vi "OAT Manually Labeled Polar Plot.vi"(0 "picture":picture, 1 "picture \ndimensions (w,h)":cluster{"width":i16, "height":i16}, 2 "polar settings":T3={"polar attributes"={"maximum"=0.0, "minimum"=0.0, "clip to min"=FALSE, "log"=FALSE, "grid color"=3381657, "plot color"=16711680, "fmt and prec"={"format"=enum."Decimal", "precision"=1}, "visible section"=8}, "desired font(Application)"=enum."Application Font", "[user-specified font]"={"Font Name:"="", "Size"=0, "Strikeout?"=FALSE, "Italic?"=FALSE, "Underline?"=FALSE, "Outline?"=FALSE, "Shadow?"=FALSE, "Bold?"=FALSE}} {"polar attributes"."minimum" format="%.2f"; "polar attributes"."maximum" format="%.2f"}, 3 "cursor attributes":T6={"layout color"=852223, "active color"=16740820, "precision"=2, "BG transparent? (T)"=FALSE, "radius"=2}, 5 "magnitude":cluster{"X":dbl[], "Y":dbl[]} {"Y" format="%.2f"; "X" format="%.2f"}, 7 "phase lag(rad)":cluster{"X":dbl[], "Y":dbl[]} {"Y" format="%.2f"; "X" format="%.2f"}, 11 "error in (no error)":errorcluster, 12 "rotating settings":T2 {"shaft rotating direction" items=["CW", "CCW"]}, 13 "phase setting":T1) -> (4 "new picture":picture, 10 "Cursor List [EU Position] Out":T4(array[cluster]) {"Location"."Y" format="%.2f"; "Location"."X" format="%.2f"}, 15 "error out":errorcluster)   [LabVIEW 2017]
doc: "Draws a polar plot on a picture control that you can interactively label."
uses:
  <vilib>/addons/Sound and Vibration/Order Analysis/Backward Compatibility/SubVIs/OAT Polar Cursor Attributes.ctl
  <vilib>/addons/Sound and Vibration/Order Analysis/_OAT State Machine/OAT State Machine Generate Events for Booleans.vi
  <vilib>/addons/Sound and Vibration/Order Analysis/_OAT State Machine/OAT State Machine Generate Event for Numeric.vi
  <vilib>/addons/Sound and Vibration/Order Analysis/_OAT State Machine/OAT State Machine Generate Events for Numerics.vi
panel:
  in  "cursor":T5={"Name"="", "Color"=0, "Hair Style"=4, "Point Style"=2, "Name Visible"=TRUE, "Trackable"=TRUE, "Lock Style"=2, "Plot Number"=0, "Marker Index"=0, "Location"={"X"=0.5, "Y"=0.5}} {"Location"."Y" format="%.2f"; "Location"."X" format="%.2f"}
  in  "exit":bool
  in  "del cursor":bool
  in  "add cursor":bool
  out "XY Graph":cluster{"X":dbl[], "Y":dbl[]}(graph)
  out "polar plot":picture
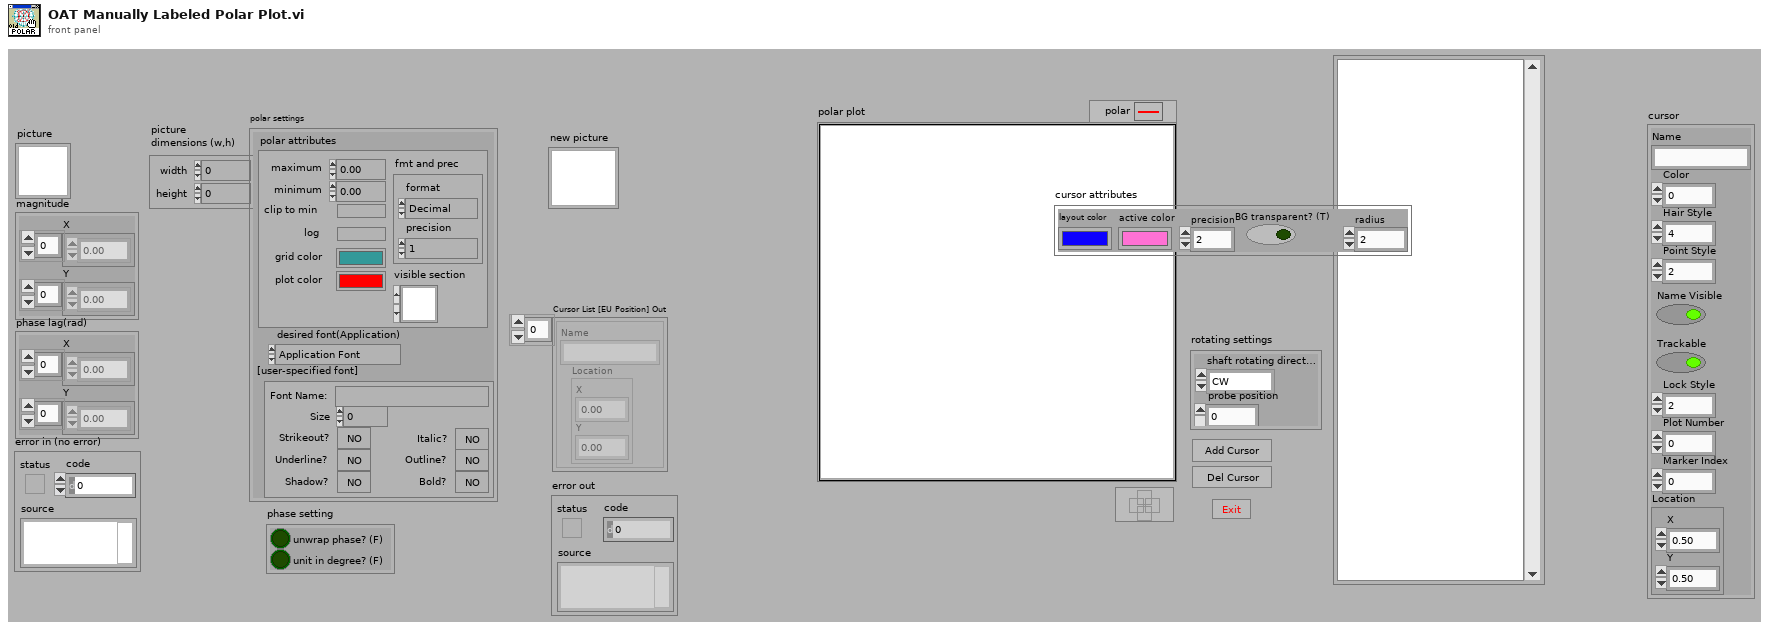
[diagram p1: front panel]
types:
  T1 = cluster{"unwrap phase? (F)":bool, "unit in degree? (F)":bool}
  T2 = cluster{"shaft rotating direction":u16, "probe position":u16}
  T3 = cluster{"polar attributes":cluster{"maximum":dbl, "minimum":dbl, "clip to min":bool, "log":bool, "grid color":u32, "plot color":u32, "fmt and prec":cluster{"format":enum8{"Decimal", "Scientific", "Engineering", "Binary", "Octal", "Hex"}, "precision":u8}, "visible section":u16}, "desired font(Application)":enum16{"User-specified Font", "Application Font", "System Font", "Dialog Font"}, "[user-specified font]":cluster{"Font Name:":string, "Size":i16, "Strikeout?":bool, "Italic?":bool, "Underline?":bool, "Outline?":bool, "Shadow?":bool, "Bold?":bool}}
  T4 = cluster{"Name":string, "Location":cluster{"X":dbl, "Y":dbl}}[]
  T5 = cluster{"Name":string, "Color":u32, "Hair Style":u8, "Point Style":u8, "Name Visible":bool, "Trackable":bool, "Lock Style":u32, "Plot Number":u32, "Marker Index":i32, "Location":cluster{"X":dbl, "Y":dbl}}
  T6 = typedef "OAT Polar Cursor Attributes.ctl" = cluster{"layout color":u32, "active color":u32, "precision":i16, "BG transparent? (T)":bool, "radius":i16}
  T7 = cluster{"Name":string, "Color":u32, "Hair Style":u8, "Point Style":u8, "Name Visible":bool, "Trackable":bool, "Lock Style":u32, "Plot Number":u32, "Marker Index":i32, "Location":cluster{"X":dbl, "Y":dbl}}[]
  T8 = cluster{"pixel center":cluster{"x":i16, "y":i16}, "scale factors":cluster{"a":dbl, "b":dbl, "log?":bool}, "grid color":u32, "start angle":dbl, "end angle":dbl, "tick length":i16, "pixel radius":i32}
  T9 = typedef "LVBoundsTypeDef.ctl" = cluster{"Width":u32, "Height":u32}
  T10 = cluster{"Name":string, "Color":u32, "Style":u8, "Point Style":u8, "Name Visible":bool, "Allow Drag":bool, "Lock Style":u32, "Plot":u32, "Index":i32, "Position":cluster{"X":dbl, "Y":dbl}}[]
  T11 = cluster{"Name":string, "Color":u32, "Style":u8, "Point Style":u8, "Name Visible":bool, "Allow Drag":bool, "Lock Style":u32, "Plot":u32, "Index":i32, "Position":cluster{"X":dbl, "Y":dbl}}
  T12 = cluster{"Name":string, "Location":cluster{"mag":dbl, "phase":dbl}}[]
  T13 = cluster{"maximum":dbl, "minimum":dbl, "clip to min":bool, "log":bool, "grid color":u32, "plot color":u32, "fmt and prec":cluster{"format":enum8{"Decimal", "Scientific", "Engineering", "Binary", "Octal", "Hex"}, "precision":u8}, "visible section":u16}
  T14 = cluster{"polar settings":cluster{"polar attributes":cluster{"maximum":dbl, "minimum":dbl, "clip to min":bool, "log":bool, "grid color":u32, "plot color":u32, "fmt and prec":cluster{"format":enum8{"Decimal", "Scientific", "Engineering", "Binary", "Octal", "Hex"}, "precision":u8}, "visible section":u16}, "desired font(Application)":enum16{"User-specified Font", "Application Font", "System Font", "Dialog Font"}, "[user-specified font]":cluster{"Font Name:":string, "Size":i16, "Strikeout?":bool, "Italic?":bool, "Underline?":bool, "Outline?":bool, "Shadow?":bool, "Bold?":bool}}, "Draw Area Size":T9, "grid measurements out":cluster{"pixel center":cluster{"x":i16, "y":i16}, "scale factors":cluster{"a":dbl, "b":dbl, "log?":bool}, "grid color":u32, "start angle":dbl, "end angle":dbl, "tick length":i16, "pixel radius":i32}}
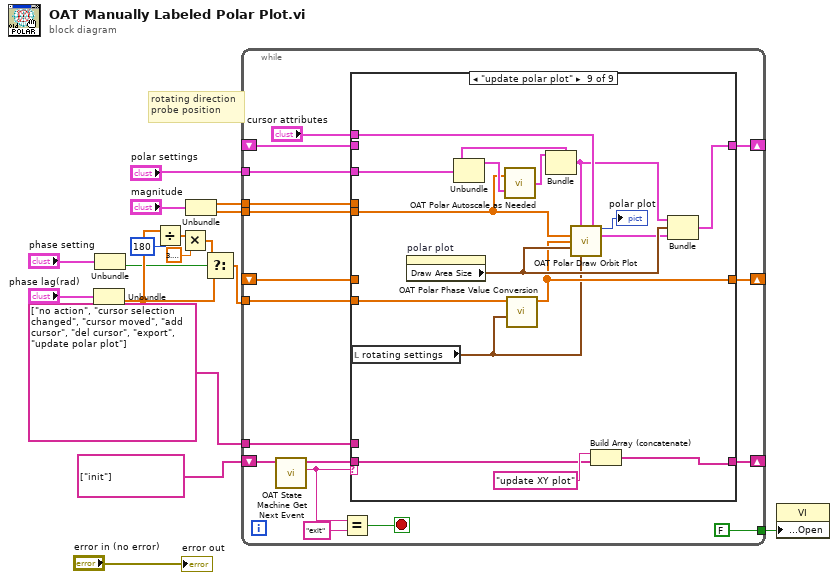
[diagram p0: block diagram]
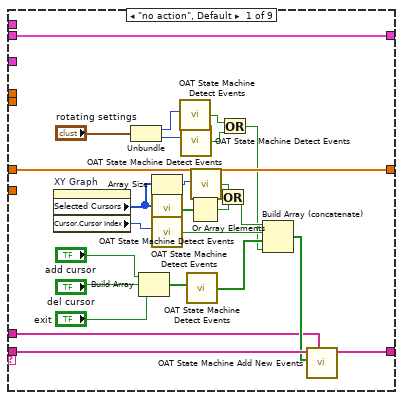
[diagram p2: hidden frame]
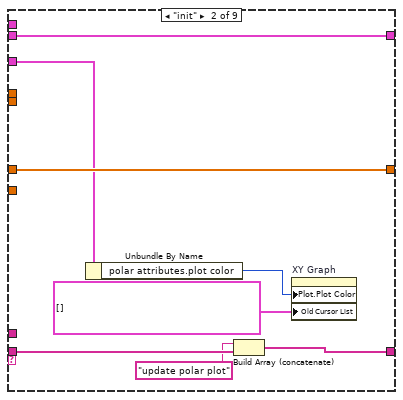
[diagram p3: hidden frame]
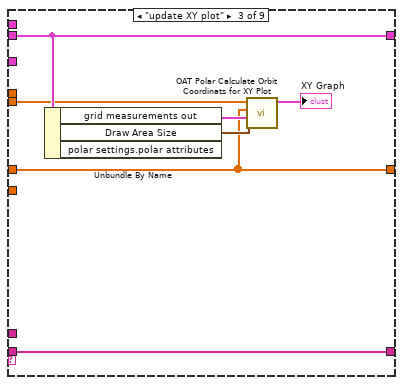
[diagram p4: hidden frame]
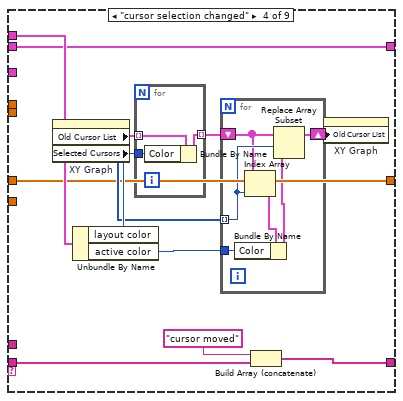
[diagram p5: hidden frame]
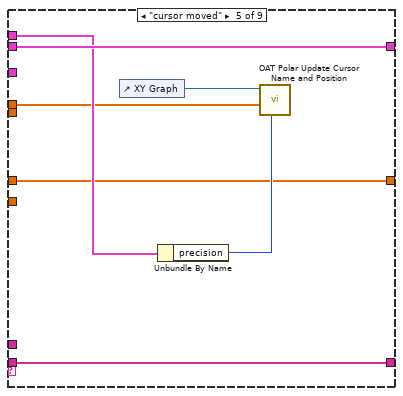
[diagram p6: hidden frame]
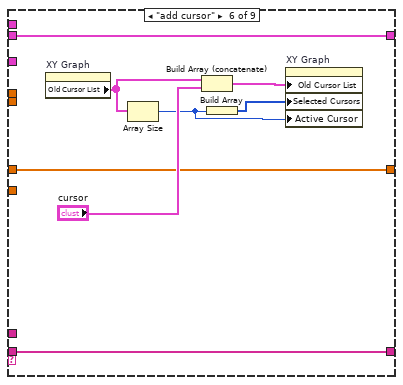
[diagram p7: hidden frame]
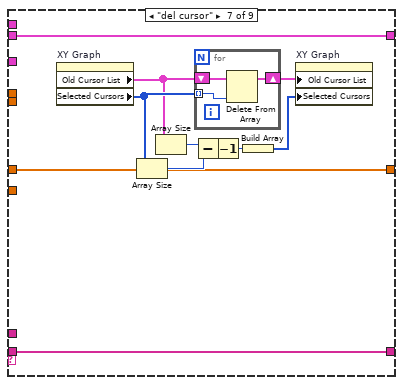
[diagram p8: hidden frame]
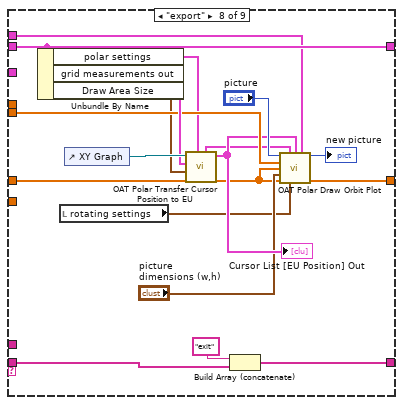
[diagram p9: hidden frame]
diagram:
  # "rotating direction\nprobe position"
  n1 = Unbundle("phase lag(rad)") -> ("Y"=w3:dbl[])  [unwired: 1 out]
  n2 = Unbundle("phase setting") -> ("unit in degree? (F)"=w1:bool)  [unwired: 1 out]
  n3 = Divide(x=w3, y=180) -> (x/y=w6:dbl[])
  n4 = Multiply(x=w6, y=3.141592653589793) -> (x*y=w4:dbl[])
  n5 = Unbundle("magnitude") -> ("X"=w9:dbl[], "Y"=w10:dbl[])
  n6 = Select(t=w4, s=w1, f=w3) -> (s? t:f=w2:dbl[])
  n7 = while {
    shift-left: _ -> [w26]
    shift-right: [w27] -> _
    tunnel: string[] ["no action", "cursor selection changed", "cursor moved", "add cursor", "del cursor", "export", "update polar plot"] ("Event Queue Out") -> [w28]
    shift-left: string[] ["init"] ("Event Queue Out") -> [w34]
    shift-right: [w32] -> _
    tunnel: w10 -> [w24]
    tunnel: w9 -> [w23]
    tunnel: [FALSE] -> w8
    shift-right: [w20] -> _
    shift-left: _ -> [w21]
    tunnel: w2 -> [w19]
    tunnel: "polar settings" -> [w18]
    stop <- w29 stop-if-true
    n8 = call <vilib>:"OAT State Machine Get Next Event.vi"("event queue in"=w34) -> ("next event"=w31:string, "event queue out"=w33:string[])  [unwired: 5 in]
    n9 = Equal?(x=w31, y="exit") -> (x = y?=w29:bool)
    n10 = case shown="\"update polar plot\"" w31 {
      tunnel: w33 -> [w59 w67 w74 w82 w102 w109 w121 w140 w150]
      tunnel: [w58 w65 w74 w81 w102 w109 w121 w139 w149] -> w32
      tunnel: w28 -> [w54 _ _ _ _ _ _ _ _]
      tunnel: "cursor attributes" -> [_ _ _ w85 w99 _ _ w133 w155]
      tunnel: [w49 w63 w73 w76 w100 w107 w112 w138 w152] -> w27
      tunnel: w26 -> [w49 w63 w73 w76 w100 w107 w112 w138 _]
      tunnel: w24 -> [_ _ w70 _ _ _ _ w132 w143]
      tunnel: w23 -> [_ _ _ _ w97 _ _ _ _]
      tunnel: w21 -> [w41 w62 w68 w75 w96 w104 w111 w127 _]
      tunnel: [w41 w62 w68 w75 w96 w104 w111 w127 w144] -> w20
      tunnel: w19 -> [_ _ _ _ _ _ _ _ w145]
      tunnel: w18 -> [_ w60 _ _ _ _ _ _ w147]
      frame "no action", Default {
        n11 = property on="XY Graph" class="XYGraph (strict)"() -> ("Selected Cursors"=w53:u32[], "Cursor.Cursor Index"=w43:i32)  [unwired: 2 in, 2 out]
        n12 = Unbundle("rotating settings") -> ("shaft rotating direction"=w36:u16, "probe position"=w35:u16)
        n13 = Build Array("add cursor", "del cursor", "exit") -> (w45:bool[])
        n14 = Array Size(array=w53) -> (size(s)=w44:i32)
        n15 = call-poly <vilib>:"OAT State Machine Detect Events.vi"("Numerics"=w53) -> ("Event Found?"=w57:bool[])  [unwired: 7 in]
        n16 = call-poly <vilib>:"OAT State Machine Detect Events.vi"("Numeric"=w43) -> ("Event"=w42:bool)  [unwired: 7 in]
        n17 = call-poly <vilib>:"OAT State Machine Detect Events.vi"("Numeric"=w36) -> ("Event"=w40:bool)  [unwired: 7 in]
        n18 = call-poly <vilib>:"OAT State Machine Detect Events.vi"("Numeric"=w35) -> ("Event"=w39:bool)  [unwired: 7 in]
        n19 = call-poly <vilib>:"OAT State Machine Detect Events.vi"("Booleans"=w45) -> ("Event Found?"=w56:bool[])  [unwired: 7 in]
        n20 = Or Array Elements(Boolean array=w57) -> (logical OR=w51:bool)
        n21 = call-poly <vilib>:"OAT State Machine Detect Events.vi"("Numeric"=w44) -> ("Event"=w52:bool)  [unwired: 7 in]
        n22 = Or(x=w52, y=w51) -> (x .or. y?=w50:bool)
        n23 = Or(x=w40, y=w39) -> (x .or. y?=w38:bool)
        n24 = Build Array (concatenate)(w50, w42, w56, w38) -> (w55:bool[])
        n25 = call <vilib>:"OAT State Machine Add New Events.vi"("Event Names"=w54, "New Events"=w55, "Event Queue In"=w59) -> ("Event Queue Out"=w58:string[])  [unwired: 8 in]
      }
      frame "init" {
        n26 = Unbundle By Name(w60) -> ("polar attributes.plot color"=w61:u32)
        n27 = Build Array (concatenate)("update polar plot", w67) -> (w65:string[])
        n28 = property on="XY Graph" class="XYGraph (strict)"("Plot.Plot Color"=w61, "Old Cursor List"=T7 [] ("Cursor List")) -> ()  [unwired: 2 in, 2 out]
      }
      frame "update XY plot" {
        n29 = Unbundle By Name(w73) -> ("grid measurements out"=w72:T8, "Draw Area Size"=w71:T9)  [unwired: 1 out]
        n30 = call <vilib>:"OAT Polar Calculate Orbit Coordinats for XY Plot.vi"("picture dimensions (w,h)"=w71, "grid measurements"=w72, "phases"=w68, "magnitudes"=w70) -> ("orbit for XY plot"=→"XY Graph":cluster{"X":dbl[], "Y":dbl[]})  [unwired: 7 in]
      }
      frame "cursor selection changed" {
        n31 = property on="XY Graph" class="XYGraph (strict)"() -> ("Old Cursor List"=w86:T10, "Selected Cursors"=w83:u32[])  [unwired: 2 in, 2 out]
        n32 = Unbundle By Name(w85) -> ("layout color"=w84:u32, "active color"=w78:u32)
        n33 = for {
          tunnel: w86 -> [w95] mode=indexing
          tunnel: w84 -> [w94]
          tunnel: [w93] -> w79 mode=indexing
          n34 = Bundle By Name(cluster=w95, "Color"=w94) -> (w93:T11)
        }
        n35 = for {
          tunnel: w83 -> [w92] mode=indexing
          shift-right: [w90] -> w77
          shift-left: w79 -> [w91]
          tunnel: w78 -> [w89]
          n36 = Index Array(array=w91, index=w92) -> (element=w88:T11)
          n37 = Bundle By Name(cluster=w88, "Color"=w89) -> (w87:T11)
          n38 = Replace Array Subset(array=w91, new element=w87, index=w92) -> (w90:T10)
        }
        n39 = Build Array (concatenate)("cursor moved", w82) -> (w81:string[])
        n40 = property on="XY Graph" class="XYGraph (strict)"("Old Cursor List"=w77) -> ()  [unwired: 2 in, 2 out]
      }
      frame "cursor moved" {
        n41 = control-ref of="XY Graph"() -> (w101:refnum<vi>)
        n42 = Unbundle By Name(w99) -> ("precision"=w98:i16)
        n43 = call <vilib>:"OAT Polar Update Cursor Name and Position.vi"("precision (2)"=w98, "X"=w97, "XY Graph"=w101) -> ()  [unwired: 8 in, 1 out]
      }
      frame "add cursor" {
        n44 = property on="XY Graph" class="XYGraph (strict)"() -> ("Old Cursor List"=w103:T10)  [unwired: 2 in, 2 out]
        n45 = Array Size(array=w103) -> (size(s)=w105:i32)
        n46 = Build Array (concatenate)(w103, "cursor") -> (w110:T7)
        n47 = Build Array(w105) -> (w106:i32[])
        n48 = property on="XY Graph" class="XYGraph (strict)"("Old Cursor List"=w110, "Selected Cursors"=w106, "Active Cursor"=w105) -> ()  [unwired: 2 in, 2 out]
      }
      frame "del cursor" {
        n49 = property on="XY Graph" class="XYGraph (strict)"() -> ("Old Cursor List"=w117:T10, "Selected Cursors"=w120:u32[])  [unwired: 2 in, 2 out]
        n50 = Array Size(array=w120) -> (size(s)=w118:i32)
        n51 = Array Size(array=w117) -> (size(s)=w119:i32)
        n52 = Subtract(x=w119, y=w118) -> (x-y=w115:i32)
        n53 = for {
          tunnel: w120 -> [w124] mode=indexing
          shift-right: [w122] -> w116
          shift-left: w117 -> [w123]
          n54 = Delete From Array(array=w123, index=w124) -> (array with subset deleted=w122:T10)  [unwired: 1 in, 1 out]
        }
        n55 = Decrement(x=w115) -> (x-1=w113:i32)
        n56 = Build Array(w113) -> (w114:i32[])
        n57 = property on="XY Graph" class="XYGraph (strict)"("Old Cursor List"=w116, "Selected Cursors"=w114) -> ()  [unwired: 2 in, 2 out]
      }
      frame "export" {
        n58 = Unbundle By Name(w138) -> ("polar settings"=w126:T3, "grid measurements out"=w134:T8, "Draw Area Size"=w131:T9)
        n59 = local read "rotating settings"() -> (w125:T2)
        n60 = control-ref of="XY Graph"() -> (w135:refnum<vi>)
        n61 = call <vilib>:"OAT Polar Transfer Cursor Position to EU.vi"("polar settings"=w126, "picture \ndimensions (w,h)"=w131, "grid measurements"=w134, "XY Graph"=w135) -> ("Cursor List (EU position]"=w130:T12, "polar settings out"=w128:T3)  [unwired: 6 in]
        "Cursor List [EU Position] Out" <- w130
        n62 = Build Array (concatenate)("exit", w140) -> (w139:string[])
        n63 = call <vilib>:"OAT Polar Draw Orbit Plot.vi"("picture"="picture", "polar settings"=w128, "Cursor List (EU position]"=w130, "cursor attributes"=w133, "magnitudes (even angular)"=w132, "phases"=w127, "picture \ndimensions (w,h)"="picture \ndimensions (w,h)", "channel settings"=w125) -> ("picture out"=→"new picture":picture)  [unwired: 6 in, 1 out]
      }
      frame "update polar plot" {
        n64 = local read "rotating settings"() -> (w142:T2)
        n65 = property on="polar plot" class="Pict"() -> ("Draw Area Size"=w157:T9)  [unwired: 2 in, 2 out]
        n66 = Unbundle(w147) -> ("polar attributes"=w154:T13)  [unwired: 2 out]
        n67 = call <vilib>:"OAT Polar Autoscale as Needed.vi"("polar attributes"=w154, "magnitudes (even angular)"=w143) -> ("polar attributes"=w153:T13)
        n68 = call <vilib>:"OAT Polar Phase Value Conversion.vi"("channel settings"=w142, "phases in"=w145) -> ("phases out"=w144:dbl[])  [unwired: 9 in]
        n69 = Bundle(cluster=w147, "polar attributes"=w153) -> (w146:T3)  [unwired: 2 in]
        n70 = call <vilib>:"OAT Polar Draw Orbit Plot.vi"("polar settings"=w146, "cursor attributes"=w155, "magnitudes (even angular)"=w143, "phases"=w144, "picture \ndimensions (w,h)"=w157, "channel settings"=w142) -> ("picture out"=→"polar plot":picture, "grid measurements out"=w156:T8)  [unwired: 8 in]
        n71 = Build Array (concatenate)("update XY plot", w150) -> (w149:string[])
        n72 = Bundle("polar settings"=w146, "Draw Area Size"=w157, "grid measurements out"=w156) -> (w152:T14)  [unwired: 1 in]
      }
    }
  }
  n73 = property class="VI"("Front Panel Window:Open"=w8) -> ()  [unwired: 2 in, 2 out]
  "error out" <- "error in (no error)"
